vi "Digital Write Single.vi"(8 "error in (no error)":errorcluster, 9 "Digital Data":bool, 10 "Channel Index":i32, 11 "Digital Writer in":refnum<class "Digital Writer.lvclass">) -> (0 "error out":errorcluster, 3 "Digital Writer out":refnum<class "Digital Writer.lvclass">)   [LabVIEW 2024, in "DAQmx Actor.lvlib" / "Digital Writer.lvclass"]
uses:
  Digital Writer.lvclass
  C:/Users/uspoaotto/OneDrive - Oregon Tool/Desktop/working copies/DAQmxActor/src/DAQmx Actor/DAQmx Actor/DAQmx Actor.lvclass
  <vilib>/DAQmx/miscellaneous.llb/DAQmx Fill In Error Info.vi
  Digital Writer.lvclass/Digital Writer.ctl
  <vilib>/DAQmx/write.llb/DAQmx Write (Digital 1D Bool NChan 1Samp 1Line).vi
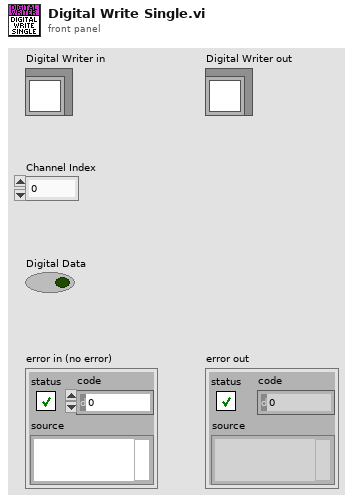
[diagram p1: front panel]
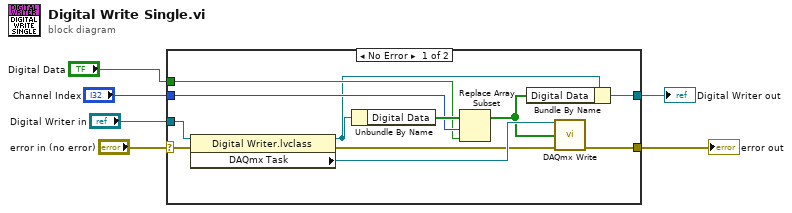
[diagram p0: block diagram]
diagram:
  n1 = case shown="No Error" "error in (no error)" {
    selector: "error in (no error)" -> [w16 w19]
    tunnel: [w15 w19] -> w5
    tunnel: [w7 w18] -> w3
    tunnel: "Digital Writer in" -> [w17 w18]
    tunnel: "Digital Data" -> [w10 _]
    tunnel: "Channel Index" -> [w11 _]
    frame No Error {
      n2 = property class="Digital Writer.lvclass"(reference=w17, error in=w16) -> (reference out=w9:refnum<class "Digital Writer.lvclass">, error out=w13:errorcluster, "DAQmx Task"=w14:refnum<k21>)
      n3 = Unbundle By Name(w9) -> ("Digital Data"=w12:bool[])
      n4 = Replace Array Subset(array=w12, new element=w10, index=w11) -> (w8:bool[])
      n5 = Bundle By Name(cluster=w9, "Digital Data"=w8) -> (w7:refnum<class "Digital Writer.lvclass">)
      n6 = call-poly <vilib>:"DAQmx Write.vi"("task/channels in"=w14, "data"=w8, "error in"=w13) -> ("error out"=w15:errorcluster)  [unwired: 10 in, 2 out]
    }
    frame Error {
    }
  }
  "error out" <- w5
  "Digital Writer out" <- w3
